vi "Create.vi"(8 "error in (no error)":errorcluster caption="错误输入（无错误）", 11 "InfoArray":T1[](array[typedef])) -> (0 "error out":errorcluster caption="错误输出", 3 "Gradient PieChart 输出":refnum<class "Gradient PieChart.lvclass"> caption="DNL_LabVIEW Object out")   [LabVIEW 2012, in "Picture Box Tools.lvlib" / "Gradient PieChart.lvclass"]
uses:
  Gradient PieChart.lvclass
  Info.ctl
  Gradient PieChart.lvclass/Gradient PieChart.ctl
panel:
  in  "Gradient PieChart 输入":refnum<class "Gradient PieChart.lvclass"> caption="DNL_LabVIEW Object in"
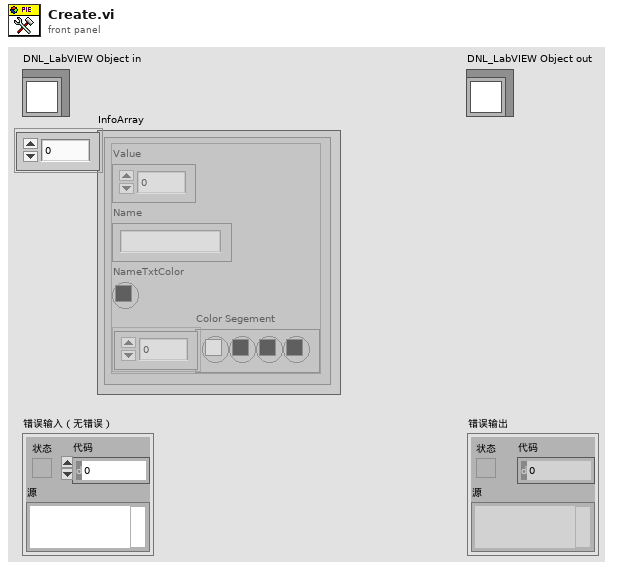
[diagram p1: front panel]
types:
  T1 = typedef "Picture Box Tools.lvlib/Gradient PieChart.lvclass/Info.ctl" = cluster{"Value":dbl, "Name":string, "NameTxtColor":u32, "Color Segement":u32[]}
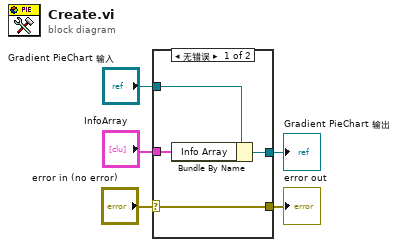
[diagram p0: block diagram]
diagram:
  n1 = case shown="无错误" "error in (no error)" {
    selector: "error in (no error)" -> [w9 w11]
    tunnel: [w9 w11] -> w4
    tunnel: [w6 w10] -> w2
    tunnel: "Gradient PieChart 输入" -> [w8 w10]
    tunnel: "InfoArray" -> [w7 _]
    frame No Error {
      n2 = Bundle By Name(cluster=w8, "Info Array"=w7) -> (w6:refnum<class "Gradient PieChart.lvclass">)
    }
    frame Error {
    }
  }
  "error out" <- w4
  "Gradient PieChart 输出" <- w2
